vi "Dashboard Main.vi"() -> ()   [LabVIEW 2013]
uses:
  <vilib>/Utility/config.llb/NI_LVConfig.lvlib
  <vilib>/Utility/config.llb/Write Key (I32).vi
  <vilib>/Rock Robotics/WPI/Dashboard/WPI_DashboardLogging Global.vi
  <vilib>/Utility/config.llb/Write Key (String).vi
  <vilib>/ErrorRing/Error Ring.xnode
  <vilib>/Analysis/NI_AALBase.lvlib
  <vilib>/Analysis/baseanly.llb/Mean (DBL).vi
  Program Files (x86)/National Instruments/LabVIEW 2013/examples/FRC/Vision/2014 Target Detection/TargetType.ctl
panel:
  out "Image Message":string="Timeout in Camera Communications"
  in  "Rec Mode":enum32{"Stop", "Record", "Playback"}(radio)
  in  "Dashboard Tab":T1(tab)
  in  "Camera Settings":T2={"Frame Rate"=30, "Compression"=30, "Size"=1} {"Frame Rate" scale=1.0..30.0; "Size" items=["640x480", "320x240", "160x120"]}
  out "MotorSliders R":cluster{"MotorSlide1":dbl, "MotorSlide2":dbl} {"MotorSlide2" scale=-1.0..1.0 scale format="%#_2e"; "MotorSlide1" scale=-1.0..1.0 scale format="%#_2e"}
  out "MotorChart R":cluster{"Numeric":dbl, "Numeric":dbl}(graph)
  out "MotorSliders L":T3 {"MotorSlide4 2" scale=0.0..14.0 scale format="%#_2e"; "MotorSlide2" scale=-1.0..1.0 scale format="%#_2e"; "MotorSlide1" scale=-1.0..1.0 scale format="%#_2e"}
  out "MotorChart L":T4(graph)
  out "JS1 Z":dbl(slide) scale=-1.0..1.0 scale format="%#_2e"
  out "Joystick 1":cluster{"X":dbl, "Y":dbl}[](graph)
  out "JS Buttons 1":T5
  out "JS2 Z":dbl(slide) scale=-1.0..1.0 scale format="%#_2e"
  out "Joystick 2":cluster{"X":dbl, "Y":dbl}[](graph)
  out "JS Buttons 2":T5
  out "Mode":T6(ring)=enum."Auto Disabled"
  out "Camera IP":string
  in  "DB Camera Config":bool
  out "fps":dbl format="%#.1g"
  out "Mbps":dbl format="%#.1g"
  out "Mbps 2":bool
  in  "Ouput Image":enum16{"Original", "Overlay", "Binary"}(ring)
  in  "Color Components":T7={"Hue"={110.0, 142.0}, "Sat"={138.0, 255.0}, "Val"={139.0, 198.0}} {"Val" scale=0.0..255.0; "Sat" scale=0.0..255.0; "Hue" scale=0.0..255.0 scale format="%#_3g"}
  in  "Std Devs":cluster{"Hue":dbl, "Sat":dbl, "Val":dbl}={"Hue"=4.0, "Sat"=6.0, "Val"=4.0}
  in  "Area Size Limit %":dbl=0.06 format="%#_13g"
  in  "Score Cutoff":dbl(slide)=54.248366013071895 scale=0.0..100.0
  out "UltrasonicRF":dbl
  out "UltrasonicLF":dbl
  out "Glass Connected":bool
  out "High Pressure":dbl
  in  "Limit":dbl
  out "Encoder FR":dbl
  out "Encoder FL":dbl
  out "Encoder RR":dbl
  out "Encoder RL":dbl
  out "Low Pressure":dbl
  in  "P":dbl=1.0
  out "Motor Outputs":dbl[](graph)
  in  "I":dbl=0.01
  in  "D":dbl
  in  "Data To Glass Type":T8(ring)
  in  "Read To Shoot?":bool=TRUE
  in  "Autonomous Enabled":bool
  in  "Reset Score":bool
  out "Side Hot":enum16{"Hot", "Not Hot"}(ring)
  out "Chance Hot":dbl
  in  "Use Left/Right":enum16{"Left", "Right"}(ring)
  in  "Test Slider":dbl(slide) scale=0.0..100.0 scale format="%#_3g"
  in  "On/Off":bool caption="Solenoid"
  in  "Test Name":u16(ring) items=["Select the test to run...", "Example Test", "-------------------------------", "List of tests is built in robot code.", "Replace with your own automated tests."]
  in  "Test Tree":string(tree)
  in  "Motor":cluster{"Value":dbl, "Enable":bool} {"Value" scale=-1.0..1.0 scale format="%#_3g"}
  out "Progress":T9 {"Test Progress" scale=0.0..100.0}
  in  "Rev/Fwd":cluster{"Forward":bool, "Reverse":bool}
  in  "Test Ring":u16(ring) items=["Auto", "Fixed indoor", "Fixed outdoor 1", "Fixed outdoor 2", "Fixed fluorescent 1", "Fixed fluorescent 2", "Hold current"]
  out "Target Info":T11(array[cluster])
  out "Tree":string(tree)
  out "Camera Image":T12(plugin-control)
  in  "Enable":bool
  # "Left"
  # "Front"
  # "Right"
  # "Battery"
  # "(Move or Just Fire)"
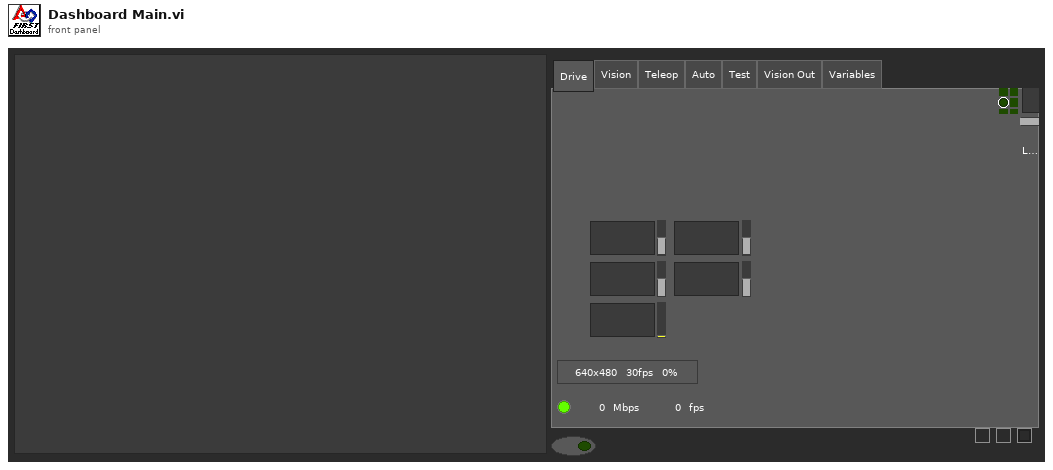
[diagram p1: front panel]
types:
  T1 = enum32{"Drive", "Vision", "Teleop", "Auto", "Test", "Vision Out", "Variables"}
  T2 = cluster{"Frame Rate":i32, "Compression":i32, "Size":u16}
  T3 = cluster{"MotorSlide1":dbl, "MotorSlide2":dbl, "MotorSlide4 2":dbl}
  T4 = cluster{"Numeric":dbl, "Numeric":dbl, "Battery":sgl}
  T5 = cluster{bool, bool, bool, bool, bool, bool, bool, bool, bool, bool, bool, bool}
  T6 = enum8{"Tele-Op Disabled", "Tele-Op Enabled", "Auto Disabled", "Auto Enabled", "Test Disabled", "Test Enabled", ""}
  T7 = cluster{"Hue":cluster{dbl, dbl}, "Sat":cluster{dbl, dbl}, "Val":cluster{dbl, dbl}}
  T8 = enum16{"Text (00)", "Shoot Status (01)", "Shoot Dist. (02)", "Pressure (03)", "Feed Dist. (04)", "Shutdown (99)"}
  T9 = cluster{"Test Progress":u8, "Test Progress Text":string}
  T10 = typedef "TargetType.ctl" = enum16{"Not Hot", "Hot"}
  T11 = cluster{"Scores":cluster{"Total":dbl, "Left":dbl, "Right":dbl, "Ratio":dbl, "Vertical":dbl, "index":i32, "State":T10}, "Verticals":cluster{"Horizontal?":bool, "Aspect Score":dbl, "Rect Score":dbl, cluster{"Left":dbl, "Top":dbl, "Right":dbl, "Bottom":dbl}, "Equiv H":dbl, "Equiv V":dbl}, "Horizontals":cluster{"Horizontal?":bool, "Aspect Score":dbl, "Rect Score":dbl, cluster{"Left":dbl, "Top":dbl, "Right":dbl, "Bottom":dbl}, "Equiv H":dbl, "Equiv V":dbl}, "Distance ft":dbl, "Center":cluster{"X":dbl, "Y":dbl}}[]
  T12 = typedef "IMAQ Image.ctl" = refnum<image>
  T13 = enum32{"Drive", "Operation", "Auto", "Test", "Checklist", "Variables"}
  T14 = typedef "Image Type" = u32
  T15 = cluster{"Digital Inputs":bool[], "Digital Outputs":bool[]}
  T16 = cluster{"Competition mode":bool, "Robot Link":bool, "Autonomous":bool, "Enabled":bool, "E-Stop":bool, "Simulated":bool, "TestMode":bool, "Docked Window":bool}
  T17 = cluster{"Boolean Array[0]":bool, "Boolean Array[1]":bool, "Boolean Array[2]":bool, "Boolean Array[3]":bool, "Boolean Array[4]":bool, "Boolean Array[5]":bool, "Boolean Array[6]":bool, "Boolean Array[7]":bool, "Boolean Array[8]":bool, "Boolean Array[9]":bool, "Boolean Array[10]":bool, "Boolean Array[11]":bool}
  T18 = typedef "NI_LVConfig.lvlib/Config Data RefNum.ctl" = refnum<k1>
  T19 = cluster{"Image Size":bool, "Image Type":bool, "Pixel Value":bool, "ROI Information":bool, "Zoom Factor":bool}
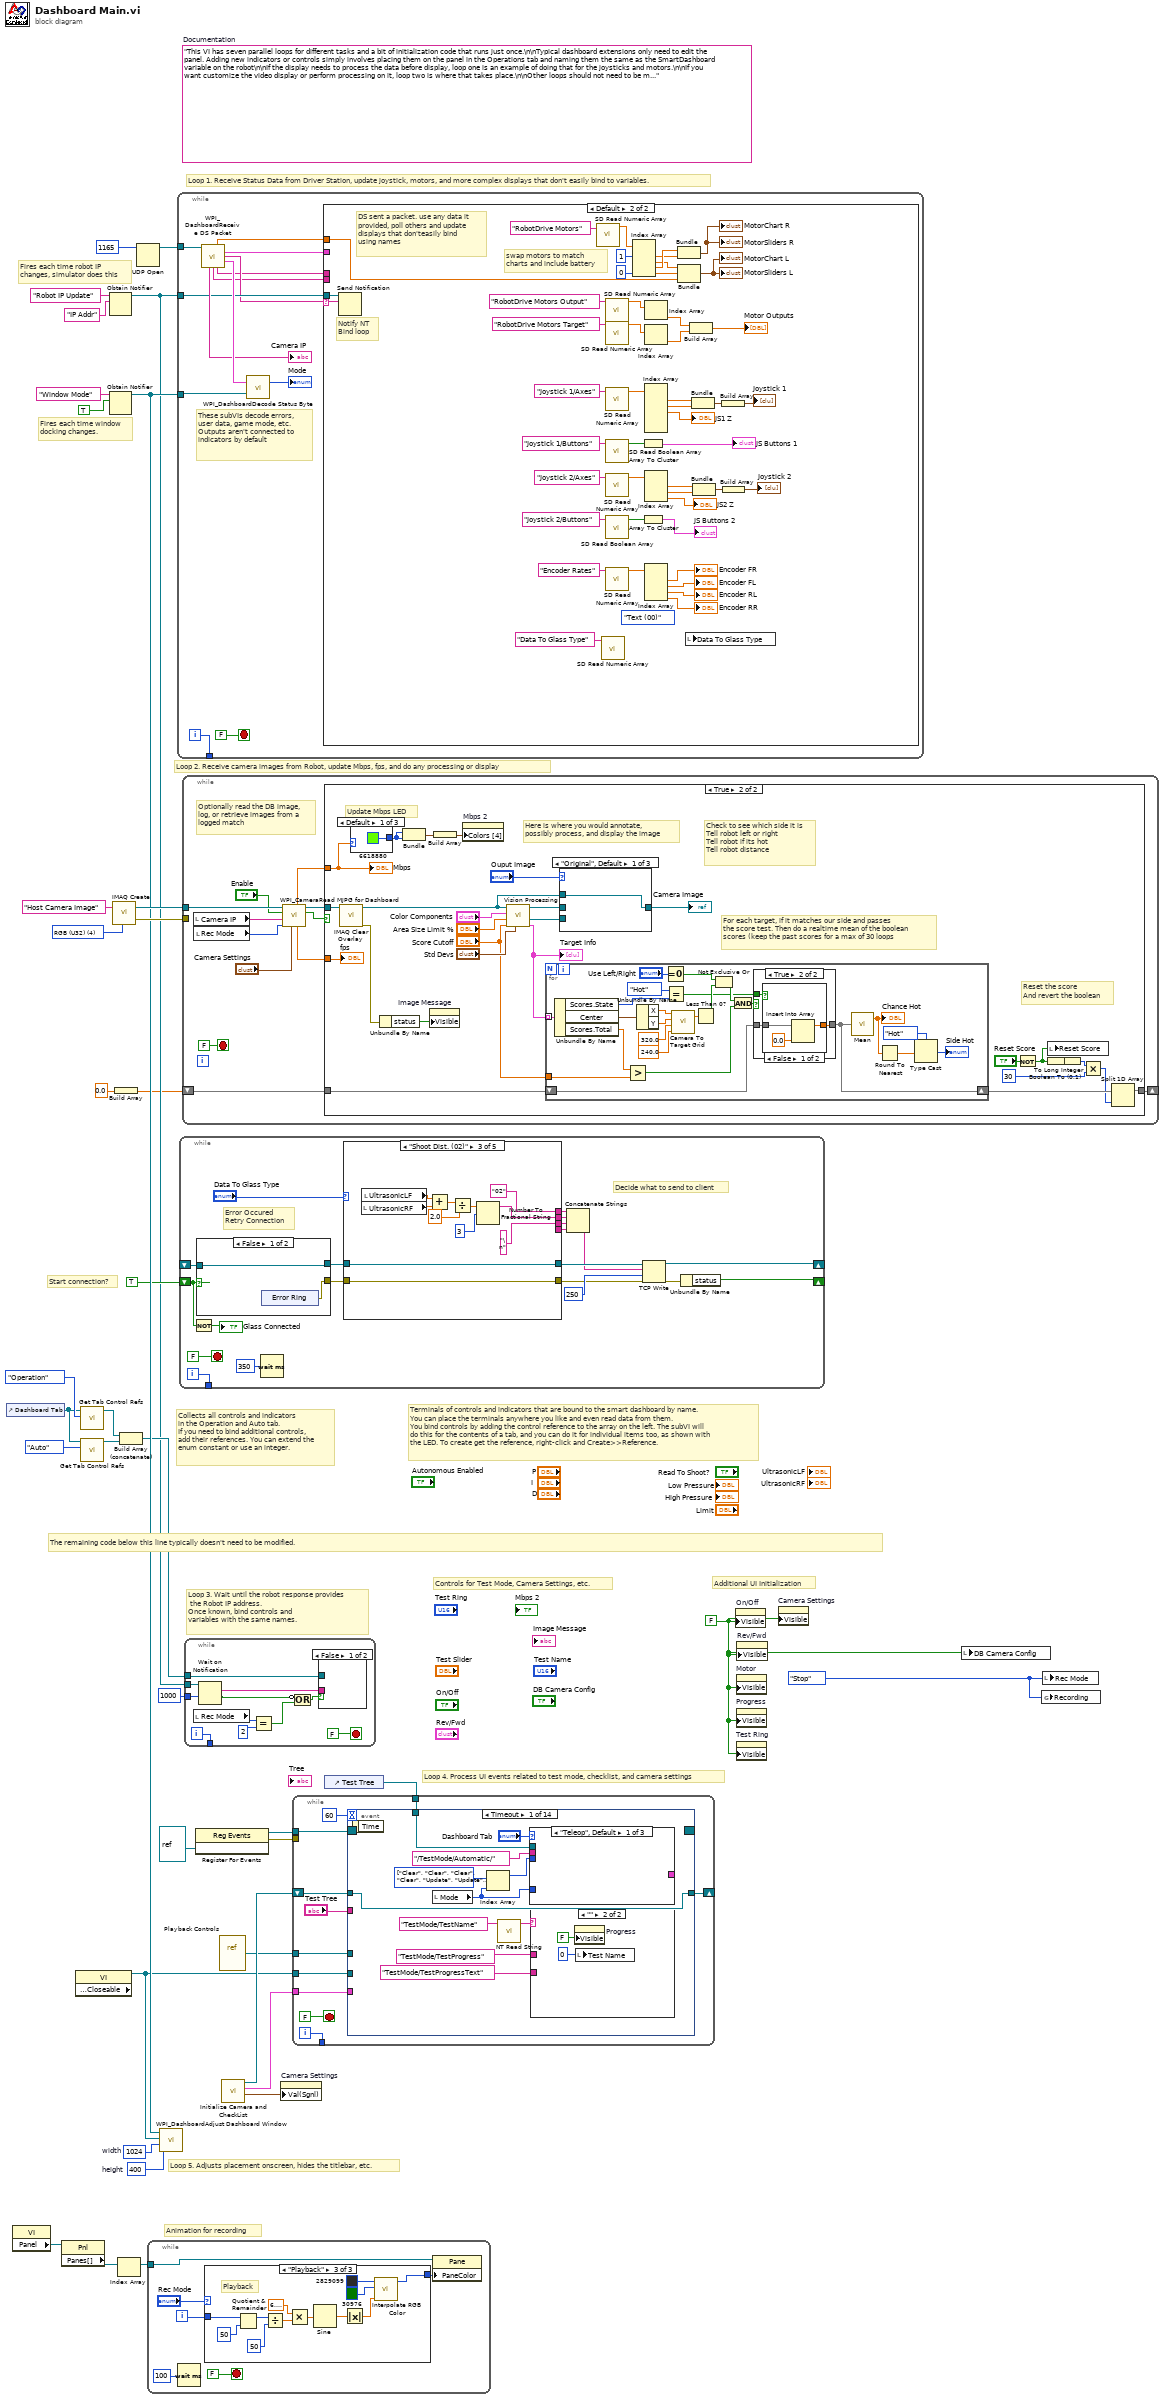
[diagram p0: block diagram]
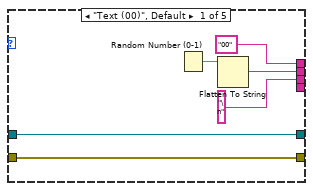
[diagram p2: hidden frame]
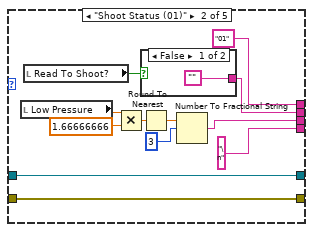
[diagram p3: hidden frame]
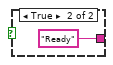
[diagram p4: hidden frame]
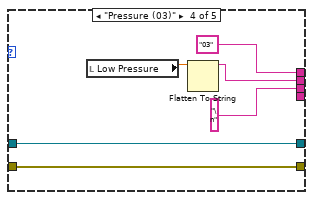
[diagram p5: hidden frame]
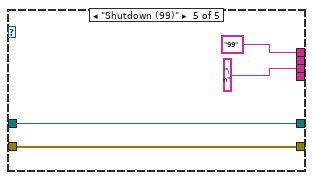
[diagram p6: hidden frame]
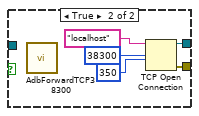
[diagram p7: hidden frame]
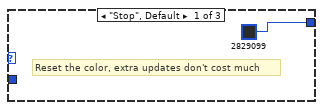
[diagram p8: hidden frame]
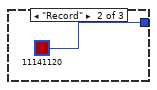
[diagram p9: hidden frame]
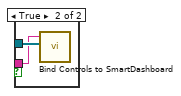
[diagram p10: hidden frame]
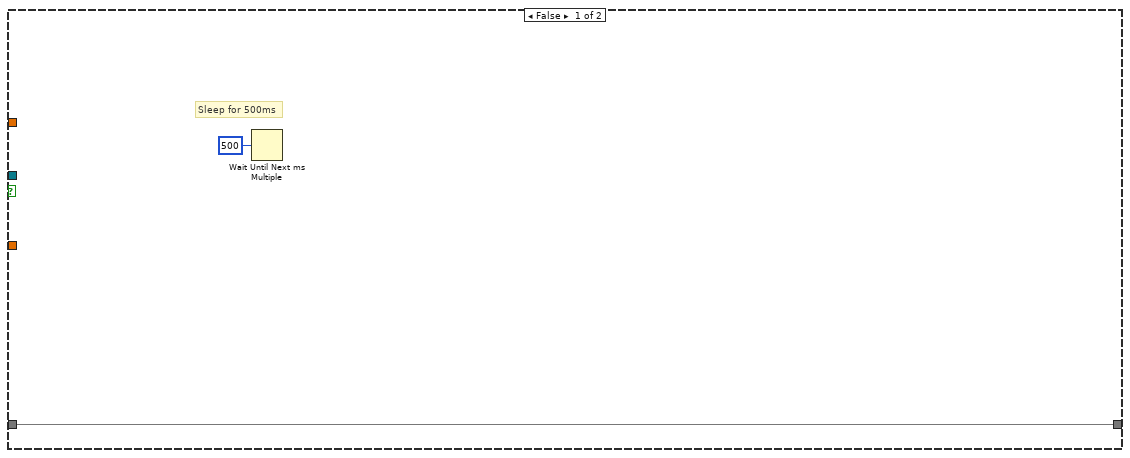
[diagram p11: hidden frame]
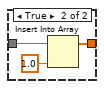
[diagram p13: hidden frame]
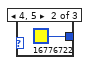
[diagram p16: hidden frame]
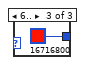
[diagram p17: hidden frame]
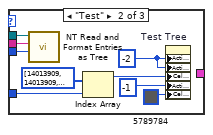
[diagram p18: hidden frame]
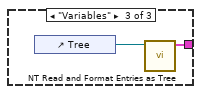
[diagram p19: hidden frame]
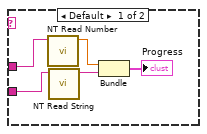
[diagram p20: hidden frame]
diagram:
  w11 = enum32{"Stop", "Record", "Playback"}."Stop" ("Rec Mode")
  w13 = 400  # height
  w14 = 1024  # width
  w27 = FALSE ("Visible")
  (unwired) "This VI has seven parallel loops for different tasks and a bit of initialization code that runs just once.\n\nTypical dashboard extensions only need to edit the panel. Adding new indicators or controls simply involves placing them on the panel in the Operations tab and naming them the same as the SmartDashboard variable on the robot\n\nIf the display needs to process the data before display, loop one is an example of doing that for the joysticks and motors.\n\nIf you want customize the video display or perform processing on it, loop two is where that takes place.\n\nOther loops should not need to be modified. They are pretty standard, and document the task they perform."  # Documentation
  w36 = T14 4 items=["Grayscale (U8)", "Grayscale (I16)", "Grayscale (SGL)", "Complex (CSG)", "RGB (U32)", "HSL (U32)", "RGB (U64)"] ("Image Type")
  # "Start connection?"
  # "Controls for Test Mode, Camera Settings, etc."
  # "Additional UI Initialization"
  # "Animation for recording"
  # "Fires each time robot IP\nchanges, simulator does this"
  # "Fires each time window\ndocking changes."
  # "Collects all controls and indicators\nin the Operation and Auto tab.\nIf you need to bind additional controls,\nadd their references. You can extend the\nenum constant or use an integer."
  # "The remaining code below this line typically doesn't need to be modified."
  # "Loop 4. Process UI events related to test mode, checklist, and camera settings"
  # "Terminals of controls and indicators that are bound to the smart dashboard by name.\nYou can place the terminals anywhere you like and even read data from them.\nYou bind controls by adding the control reference to the array on the left. The subVI will\ndo this for the contents of a tab, and you can do it for individual items too, as shown with\nthe LED. To create get the reference, right-click and Create>>Reference."
  # "Loop 3. Wait until the robot response provides\n the Robot IP address.\nOnce known, bind controls and\nvariables with the same names."
  # "Loop 5. Adjusts placement onscreen, hides the titlebar, etc."
  # "Loop 1. Receive Status Data from Driver Station, update joystick, motors, and more complex displays that don't easily bind to variables."
  # "Loop 2. Receive camera images from Robot, update Mbps, fps, and do any processing or display"
  n1 = control-ref of="Dashboard Tab"() -> (w9:refnum<vi>)
  n2 = property class="VI"() -> ("Panel"=w21:refnum<vi>)  [unwired: 2 in, 2 out]
  n3 = property class="Pnl"(reference=w21) -> ("Panes[]"=w22:refnum<vi>[])  [unwired: 1 in, 2 out]
  n4 = property class="VI" props=["Front Panel.Closeable"]() -> (reference out=w10:refnum<vi>)  [unwired: 2 in, 2 out]
  n5 = call <vilib>:"Get Tab Control Refs.vi"("Page Index"=T13."Operation" ("Dashboard Tab"), "TabControl in"=w9) -> ("ControlsOnPage"=w7:refnum<vi>[])  [unwired: 9 in]
  n6 = call <vilib>:"Get Tab Control Refs.vi"("Page Index"=T13."Auto" ("Dashboard Tab"), "TabControl in"=w9) -> ("ControlsOnPage"=w8:refnum<vi>[])  [unwired: 9 in]
  n7 = Obtain Notifier(name (unnamed)="Robot IP Update", notification data type="IP Addr" ("name (unnamed)")) -> (notifier out=w3:refnum<notifier>)  [unwired: 2 in, 2 out]
  n8 = Obtain Notifier(name (unnamed)="Window Mode", notification data type=TRUE) -> (notifier out=w12:refnum<notifier>)  [unwired: 2 in, 2 out]
  n9 = call "IMAQ Create"("Image Name"="Host Camera Image", "Image Type"=w36) -> ("New Image"=w34:T12, "error out"=w33:errorcluster)  [unwired: 2 in, 1 out]
  n10 = Build Array(0.0 ("element")) -> (w2:dbl[])
  n11 = Index Array(array=w22) -> (element=w20:refnum<vi>)  [unwired: 1 in]
  n12 = Build Array (concatenate)(w7, w8) -> (w6:refnum<vi>[])
  n13 = UDP Open(11:u16 1165 ("port")) -> (port=w37:refnum<k16>)  [unwired: 2 in, 4 out]
  n14 = while {
    tunnel: w20 -> [w40]
    i -> [w43]
    stop <- FALSE stop-if-true
    n15 = Wait (ms)(milliseconds to wait=u32 100) -> ()  [unwired: 1 out]
    n16 = case shown="\"Playback\"" "Rec Mode" {
      tunnel: w43 -> [_ _ w58]
      tunnel: [u32 2829099 ("Base Color") u32 11141120 ("Target Color") w47] -> w39
      frame "Stop", Default {
        # "Reset the color, extra updates don't cost much"
      }
      frame "Record" {
      }
      frame "Playback" {
        # "Playback"
        n17 = Quotient & Remainder(x=w58, y=u32 50 ("milliseconds to wait")) -> (x-y*floor(x/y)=w54:u32)  [unwired: 1 out]
        n18 = Divide(x=w54, y=u32 50 ("milliseconds to wait")) -> (x/y=w51:dbl)
        n19 = Multiply(x=6.283185307179586, y=w51) -> (x*y=w56:dbl)
        n20 = Sine(x=w56) -> (sin(x)=w55:dbl)
        n21 = Absolute Value(x=w55) -> (abs(x)=w48:dbl)
        n22 = call "Interpolate RGB Color.vi"("Proportion"=w48, "Target Color"=u32 30976, "Base Color"=u32 2829099) -> ("Result Color"=w47:u32)  [unwired: 8 in]
      }
    }
    n23 = property class="Pane"(reference=w40, "PaneColor"=w39) -> ()  [unwired: 1 in, 2 out]
  }
  n24 = call <vilib>:"WPI_DashboardAdjust Dashboard Window.vi"("height"=w13, "width"=w14, "reference in"=w10, "Notifier in"=w12) -> ()  [unwired: 8 in]
  n25 = while {
    tunnel: w37 -> [w69]
    tunnel: w3 -> [w64]
    tunnel: w12 -> [w68]
    tunnel: [w65] -> _
    i -> [w65]
    stop <- FALSE stop-if-true
    # "These subVIs decode errors, user data, game mode, etc.\nOutputs aren't connected to indicators by default"
    n26 = call <vilib>:"WPI_DashboardReceive DS Packet.vi"("Recv Socket"=w69) -> ("Battery"=w59:sgl, "Driver Station"=w60:T15, "Robot IP Address"=w63:string, "Status"=w70:T16, "Camera IP Address"=→"Camera IP":string, "Low Priority User Data"=w62:string, "High Priority User Data"=w61:string)  [unwired: 1 in, 7 out]
    n27 = call <vilib>:"WPI_DashboardDecode Status Byte.vi"("Window Mode Notifier"=w68, "Status"=w70) -> ("Mode"=→"Mode":T6)  [unwired: 1 out]
    n28 = case shown="Default" w63 {
      selector: w63 -> [_ w96]
      tunnel: w64 -> [_ w97]
      tunnel: w62 -> [_ _]
      tunnel: w61 -> [_ _]
      tunnel: w60 -> [_ _]
      tunnel: w59 -> [_ w95]
      frame "0.0.0.0" {
        # "DS not sending packets, or no robot exists yet.\nDon't poll the variables"
      }
      frame Default {
        (unwired) T8."Text (00)" ("Data To Glass Type")
        # "Notify NT\nBind loop"
        # "DS sent a packet. use any data it\nprovided, poll others and update\ndisplays that don'teasily bind\nusing names"
        # "swap motors to match\ncharts and include battery"
        n29 = Send Notification(notification=w96, notifier=w97) -> ()  [unwired: 1 in, 2 out]
        n30 = call <vilib>:"SD Read Numeric Array.vi"("Name"="RobotDrive Motors") -> ("Numeric Array"=w94:dbl[])  [unwired: 8 in, 2 out]
        n31 = call <vilib>:"SD Read Numeric Array.vi"("Name"="Data To Glass Type") -> ()  [unwired: 8 in, 3 out]
        n32 = call <vilib>:"SD Read Numeric Array.vi"("Name"="RobotDrive Motors Output") -> ("Numeric Array"=w82:dbl[])  [unwired: 8 in, 2 out]
        n33 = call <vilib>:"SD Read Numeric Array.vi"("Name"="RobotDrive Motors Target") -> ("Numeric Array"=w80:dbl[])  [unwired: 8 in, 2 out]
        n34 = call <vilib>:"SD Read Numeric Array.vi"("Name"="Joystick 1/Axes") -> ("Numeric Array"=w113:dbl[])  [unwired: 8 in, 2 out]
        n35 = call <vilib>:"SD Read Boolean Array.vi"("Name"="Joystick 1/Buttons") -> ("Boolean Array"=w115:bool[])  [unwired: 8 in, 2 out]
        n36 = call <vilib>:"SD Read Numeric Array.vi"("Name"="Joystick 2/Axes") -> ("Numeric Array"=w107:dbl[])  [unwired: 8 in, 2 out]
        n37 = call <vilib>:"SD Read Boolean Array.vi"("Name"="Joystick 2/Buttons") -> ("Boolean Array"=w106:bool[])  [unwired: 8 in, 2 out]
        n38 = call <vilib>:"SD Read Numeric Array.vi"("Name"="Encoder Rates") -> ("Numeric Array"=w75:dbl[])  [unwired: 8 in, 2 out]
        n39 = Index Array(array=w94, index #1=1, index #4=0) -> (element #1=w90:dbl, element #2=w89:dbl, element #3=w91:dbl, element #4=w86:dbl)  [unwired: 2 in]
        n40 = Array To Cluster(array=w115) -> (cluster=→"JS Buttons 1":T17)
        n41 = Array To Cluster(array=w106) -> (cluster=→"JS Buttons 2":T17)
        n42 = Index Array(array=w82) -> (element=w81:dbl)  [unwired: 1 in]
        n43 = Index Array(array=w80) -> (element=w74:dbl)  [unwired: 1 in]
        n44 = Index Array(array=w113) -> (element #1=w110:dbl, element #2=w111:dbl, element #3=→"JS1 Z":dbl)  [unwired: 6 in, 3 out]
        n45 = Index Array(array=w107) -> (element #1=w102:dbl, element #2=w101:dbl, element #3=→"JS2 Z":dbl)  [unwired: 3 in]
        n46 = Index Array(array=w75) -> (element #1=→"Encoder FR":dbl, element #2=→"Encoder FL":dbl, element #3=→"Encoder RL":dbl, element #4=→"Encoder RR":dbl)  [unwired: 4 in]
        n47 = Bundle("Numeric"=w91, "Numeric"=w90) -> (→"MotorChart R" →"MotorSliders R":cluster{"Numeric":dbl, "Numeric":dbl})  [unwired: 1 in]
        n48 = Bundle("Numeric"=w89, "Numeric"=w86, "Battery"=w95) -> (→"MotorChart L" →"MotorSliders L":T4)  [unwired: 1 in]
        n49 = local read "Data To Glass Type"() -> ()  [unwired: 1 in]
        n50 = Build Array(w81, w74) -> (→"Motor Outputs":dbl[])
        n51 = Bundle("Numeric"=w110, "Numeric"=w111) -> (w109:cluster{"Numeric":dbl, "Numeric":dbl})  [unwired: 1 in]
        n52 = Bundle("Numeric"=w102, "Numeric"=w101) -> (w103:cluster{"Numeric":dbl, "Numeric":dbl})  [unwired: 1 in]
        n53 = Build Array(w109) -> (→"Joystick 1":cluster{"Numeric":dbl, "Numeric":dbl}[])
        n54 = Build Array(w103) -> (→"Joystick 2":cluster{"Numeric":dbl, "Numeric":dbl}[])
      }
    }
  }
  n55 = while {
    tunnel: [w137] -> _
    shift-right: [w134] -> _
    shift-left: TRUE ("status") -> [w120]
    shift-right: [w133] -> _
    shift-left: _ -> [w132]
    i -> [w137]
    stop <- FALSE stop-if-true
    # "Decide what to send to client"
    # "Error Occured \nRetry Connection"
    n56 = Not(x=w120) -> (.not. x?=→"Glass Connected":bool)
    n57 = case shown="False" w120 {
      tunnel: [w181 w184] -> w127
      tunnel: [w180 w183] -> w129
      tunnel: w132 -> [w181 _]
      frame False {
        n58 = xnode "Error Ring"() -> ("error out"=w180:errorcluster)
      }
      frame True {
        n59 = call "AdbForwardTCP38300.vi"() -> ()  [unwired: 12 in]
        n60 = TCP Open Connection(address="localhost", remote port or service name=u16 38300, timeout ms (60000)=350) -> (connection ID=w184:refnum<k5>, error out=w183:errorcluster)  [unwired: 2 in]
      }
    }
    n61 = Wait (ms)(milliseconds to wait=u32 350) -> ()  [unwired: 1 out]
    n62 = case shown="\"Shoot Dist. (02)\"" "Data To Glass Type" {
      tunnel: [w143 w155 w163 w174 w178] -> w128
      tunnel: w129 -> [w143 w155 w163 w174 w178]
      tunnel: w127 -> [w142 w156 w160 w175 w179]
      tunnel: [w142 w156 w160 w175 w179] -> w126
      tunnel: ["\n" ("string") w146 "\n" ("string") "\n" ("string") "\n" ("string")] -> w124
      tunnel: ["00" ("string") "01" ("string") "02" ("string") "03" ("string") "99" ("string")] -> w123
      tunnel: [w140 w152 w162 w171 _] -> w122
      tunnel: [_ "\n" ("string") _ _ _] -> w119
      frame "Text (00)", Default {
        n63 = Random Number (0-1)() -> (number: 0 to 1=w144:dbl)
        n64 = Flatten To String(anything=w144) -> (data string=w140:string)  [unwired: 3 in, 2 out]
      }
      frame "Shoot Status (01)" {
        n65 = local read "Low Pressure"() -> (w150:dbl)
        n66 = local read "Read To Shoot?"() -> (w154:bool)
        n67 = Multiply(x=w150, y=1.66666666) -> (x*y=w149:dbl)
        n68 = case shown="False" w154 {
          tunnel: ["" "Ready"] -> w152
          frame False {
          }
          frame True {
          }
        }
        n69 = Round To Nearest(number=w149) -> (nearest integer value=w147:dbl)
        n70 = Number To Fractional String(number=w147, width (-)=i16 3) -> (F-format string=w146:string)  [unwired: 2 in]
      }
      frame "Shoot Dist. (02)" {
        n71 = local read "UltrasonicRF"() -> (w168:dbl)
        n72 = local read "UltrasonicLF"() -> (w169:dbl)
        n73 = Add(x=w169, y=w168) -> (x+y=w167:dbl)
        n74 = Divide(x=w167, y=2.0) -> (x/y=w161:dbl)
        n75 = Number To Fractional String(number=w161, width (-)=i16 3) -> (F-format string=w162:string)  [unwired: 2 in]
      }
      frame "Pressure (03)" {
        n76 = local read "Low Pressure"() -> (w173:dbl)
        n77 = Flatten To String(anything=w173) -> (data string=w171:string)  [unwired: 3 in, 2 out]
      }
      frame "Shutdown (99)" {
      }
    }
    n78 = Concatenate Strings(w123, w122, w124, w119) -> (w125:string)
    n79 = TCP Write(connection ID=w126, data in=w125, error in (no error)=w128, 9:250 ("timeout ms (25000)")) -> (connection ID out=w133:refnum<k5>, error out=w135:errorcluster)  [unwired: 1 out]
    n80 = Unbundle By Name(w135) -> ("status"=w134:bool)
  }
  n81 = while {
    tunnel: w34 -> [w198]
    tunnel: w33 -> [_]
    shift-right: [w188] -> _
    shift-left: w2 -> [w189]
    stop <- FALSE stop-if-true
    # "Optionally read the DB image,\nlog, or retrieve images from a\nlogged match"
    n82 = local read "Camera IP"() -> (w191:string)
    n83 = local read "Rec Mode"() -> (w190:enum32{"Stop", "Record", "Playback"})
    n84 = call <vilib>:"WPI_CameraRead MJPG for Dashboard.vi"("Camera Settings"="Camera Settings", "Rec Mode"=w190, "Camera IP"=w191, "Enable"="Enable", "Refnum in"=w198) -> ("Active"=w195:bool, "Refnum out"=w197:T12, "FPS"=w194:dbl, "Bandwidth (Mbps)"=w193:dbl)  [unwired: 3 in]
    n85 = case shown="True" w195 {
      tunnel: w197 -> [_ w223]
      tunnel: w193 -> [_ w222]
      tunnel: w194 -> [_ w221]
      tunnel: w189 -> [w200 w210]
      tunnel: [w200 w208] -> w188
      frame False {
        # "Sleep for 500ms"
        n86 = Wait Until Next ms Multiple(millisecond multiple=u32 500) -> ()  [unwired: 1 out]
      }
      frame True {
        # "Reset the score\nAnd revert the boolean"
        # "For each target, if it matches our side and passes\nthe score test. Then do a realtime mean of the boolean\nscores (keep the past scores for a max of 30 loops"
        # "Check to see which side it is\nTell robot left or right\nTell robot if its hot\nTell robot distance"
        # "Here is where you would annotate,\npossibly process, and display the image"
        # "Update Mbps LED"
        n87 = call "IMAQ Clear Overlay"("Image"=w223) -> ("error out"=w227:errorcluster, "Image Out"=w213:T12)  [unwired: 2 in, 7 out]
        n88 = case shown="Default" w222 {
          tunnel: [u32 6618880 ("Color Box") u32 16776722 ("Color Box") u32 16716800 ("Color Box")] -> w224
          frame Default {
          }
          frame 4, 5 {
          }
          frame 6.. {
          }
        }
        n89 = Unbundle By Name(w227) -> ("status"=w228:bool)
        n90 = Bundle("Color Box"=w224, "Color Box"=w224) -> (w226:cluster{"Color Box":u32, "Color Box":u32})  [unwired: 1 out]
        n91 = property on="Image Message" class="Str"("Visible"=w228) -> ()  [unwired: 2 in, 2 out]
        n92 = Build Array(w226) -> (w225:cluster{"Color Box":u32, "Color Box":u32}[])
        n93 = property on="Mbps 2" class="Bool (strict)"("Colors [4]"=w225) -> ()  [unwired: 2 in, 2 out]
        n94 = call "Vision Processing.vi"("Std Devs"="Std Devs", "Score Cutoff"="Score Cutoff", "Area Size Limit %"="Area Size Limit %", "Color Components"="Color Components", "Image In"=w213) -> ("Target Info"=w212:T11, "Mask"=w214:T12, "Image Out"=w215:T12)  [unwired: 4 in]
        "Target Info" <- w212
        n95 = for {
          tunnel: w212 -> [w251] mode=indexing
          tunnel: "Score Cutoff" -> [w239]
          shift-right: [w229] -> w209
          shift-left: w210 -> [w234]
          n96 = Unbundle By Name(w251) -> ("Scores.State"=w245:T10, "Center"=w252:cluster{"X":dbl, "Y":dbl}, "Scores.Total"=w240:dbl)
          n97 = Greater?(x=w240, y=w239) -> (0:w232:bool)
          n98 = Unbundle By Name(w252) -> ("X"=w250:dbl, "Y"=w249:dbl)
          n99 = Equal To 0?(x="Use Left/Right") -> (x = 0?=w242:bool)
          n100 = Equal?(x=TargetType."Hot", y=w245) -> (x = y?=w230:bool)
          n101 = call "Camera To Target Grid.vi"("Height"=240.0, "Width"=320.0, "CY"=w249, "CX"=w250) -> ("X'"=w247:dbl)  [unwired: 1 out]
          n102 = Less Than 0?(x=w247) -> (x < 0?=w243:bool)
          n103 = Not Exclusive Or(1:w243, 2:w242) -> (0:w231:bool)
          n104 = And(x=w231, y=w232) -> (x .and. y?=w233:bool)
          n105 = case shown="True" w233 {
            tunnel: w234 -> [w253 w256]
            tunnel: [w253 w255] -> w229
            tunnel: w230 -> [_ w254]
            frame False {
            }
            frame True {
              n106 = case shown="False" w254 {
                tunnel: w256 -> [w258 w262]
                tunnel: [w257 w260] -> w255
                frame False {
                  n107 = Insert Into Array(array=w258, new element=0.0 ("new element/subarray")) -> (w257:dbl[])  [unwired: 1 in]
                }
                frame True {
                  n108 = Insert Into Array(array=w262, new element=1.0 ("new element/subarray")) -> (w260:dbl[])  [unwired: 1 in]
                }
              }
            }
          }
          n109 = call-poly <vilib>:"Mean.vi"("X"=w229) -> ("mean"=w238:dbl)  [unwired: 1 out]
          "Chance Hot" <- w238
          n110 = Round To Nearest(number=w238) -> (nearest integer value=w235:dbl)
          n111 = Type Cast(type=enum16{"Hot", "Not Hot"}."Hot" ("Side Hot"), x=w235) -> (*(type *) &x=→"Side Hot":enum16{"Hot", "Not Hot"})
        }
        n112 = case shown="\"Original\", Default" "Ouput Image" {
          tunnel: [w263 w264 w265] -> w216
          tunnel: w215 -> [_ w264 _]
          tunnel: w214 -> [_ _ w265]
          tunnel: w213 -> [w263 _ _]
          frame "Original", Default {
          }
          frame "Overlay" {
          }
          frame "Binary" {
          }
        }
        "Camera Image" <- w216
        n113 = Not(x="Reset Score") -> (.not. x?=w202:bool)
        n114 = Boolean To (0,1)(Boolean=w202) -> (0, 1=w205:i16)
        n115 = local write "Reset Score"(w202) -> ()
        n116 = To Long Integer(number=w205) -> (32bit integer=w204:i32)
        n117 = Multiply(x=w204, y=30 ("index")) -> (x*y=w203:i32)
        n118 = Split 1D Array(array=w209, index=w203) -> (first subarray=w208:dbl[])  [unwired: 1 out]
        "Mbps" <- w222
        "fps" <- w221
      }
    }
  }
  n119 = while {
    tunnel: w6 -> [w279]
    tunnel: w3 -> [w277]
    tunnel: [w275] -> _
    tunnel: u32 1000 ("milliseconds to wait") -> [w274]
    i -> [w275]
    stop <- FALSE stop-if-true
    n120 = local read "Rec Mode"() -> (w270:enum32{"Stop", "Record", "Playback"})
    n121 = Wait on Notification(notifier=w277, timeout in ms (-1)=w274) -> (notification=w276:string, timed out?=w272:bool)  [unwired: 2 in, 2 out]
    n122 = Equal?(x=w270, y=u16 2 ("Rec Mode")) -> (x = y?=w271:bool)
    n123 = Compound Arithmetic op=OR(invert w272, w271) -> (w273:bool)
    n124 = case shown="False" w273 {
      tunnel: w279 -> [_ w281]
      tunnel: w276 -> [_ w280]
      frame False {
      }
      frame True {
        n125 = call <vilib>:"Bind Controls to SmartDashboard.vi"("Bound Control Refs"=w281, "Server IP Address"=w280) -> ()  [unwired: 10 in]
      }
    }
  }
  n126 = register-events(refnum<vi> refnum) -> (reference out=w18:refnum<event-registration>, error out=w17:errorcluster)  [unwired: 2 in]
  n127 = vi-ref "Playback Controls.vi"() -> (w19:refnum<vi>)
  n128 = call "Initialize Camera and CheckList.vi"() -> ("Cluster"=w25:cluster{"value":i32, "value":i32, "index":i32}, "Array"=w26:cluster{string[]}[], "File Refnum"=w24:T18)  [unwired: 9 in]
  n129 = property on="Camera Settings" class="Clust (strict)"("Val(Sgnl)"=w25) -> ()  [unwired: 2 in, 2 out]
  n130 = control-ref of="Test Tree"() -> (w23:refnum<vi>)
  n131 = while {
    tunnel: w26 -> [w289]
    shift-right: [w288] -> _
    shift-left: w24 -> [w287]
    tunnel: [w286] -> _
    tunnel: w23 -> [w285]
    tunnel: w19 -> [w284]
    tunnel: w18 -> [w283]
    tunnel: w17 -> [_]
    tunnel: w10 -> [w282]
    i -> [w286]
    stop <- FALSE stop-if-true
    n132 = event shown="[0] Timeout" {
      selector: w283 -> [_ _ _ _ _ _ _ _ _ _ _ _ _ _]
      dyn-events: [_ _ _ _ _ _ _ _ _ _ _ w503 _ _] -> _
      timeout: u32 60 ("milliseconds to wait") -> [_ _ _ _ _ _ _ _ _ _ _ _ _ _]
      tunnel: w285 -> [w299 _ _ _ _ _ _ _ _ _ _ _ _ _]
      tunnel: "Test Tree" -> [_ _ _ _ _ _ w472 w480 w482 w486 w494 _ _ _]
      tunnel: w289 -> [_ w323 _ _ w436 w466 _ _ _ _ _ _ _ _]
      tunnel: [w293 w322 w421 w426 w435 w459 w471 w478 w481 w485 w493 w505 w519 w520] -> w288
      tunnel: w287 -> [w293 w322 w421 w426 w434 w459 w471 w478 w481 w485 w493 w505 w519 w520]
      tunnel: w284 -> [_ _ _ _ _ _ _ _ _ _ _ w506 _ w523]
      tunnel: w282 -> [_ _ _ _ _ _ _ _ _ _ _ w501 _ _]
      event Timeout {
        w298 = enum16{"Update", "Clear"}[] [enum."Clear", enum."Clear", enum."Clear", enum."Clear", enum."Update", enum."Update", enum."Clear"] items=["Update", "Clear"]
        n133 = event-data() -> ()  [unwired: 1 in, 1 out]
        n134 = local read "Mode"() -> (w296:T6)
        n135 = Index Array(array=w298, index=w296) -> (element=w297:enum16{"Update", "Clear"})
        n136 = call <vilib>:"NT Read String.vi"("Name"="TestMode/TestName") -> ("String"=w302:string)  [unwired: 9 in, 1 out]
        n137 = case shown="\"Teleop\", Default" "Dashboard Tab" {
          tunnel: w299 -> [_ w312 _]
          tunnel: "/TestMode/Automatic/" ("Name Pattern") -> [_ w311 _]
          tunnel: w297 -> [_ w310 _]
          tunnel: w296 -> [_ w308 _]
          tunnel: [_ _ w314] -> _
          frame "Teleop", Default {
          }
          frame "Test" {
            w307 = -2 ("Active Item:Row Number")
            n138 = call <vilib>:"NT Read and Format Entries as Tree.vi"("Operation"=w310, "Name Pattern"=w311, "Tree Refnum"=w312) -> ()  [unwired: 7 in, 2 out]
            n139 = Index Array(array=u32[] [14013909, 14013909, 14013909, 14013909, 14013909, 16777215, 14013909], index=w308) -> (element=w306:u32)
            n140 = property on="Test Tree" class="Tree (strict)"("Active Item Row Number"=w307, "ActiveColNum"=w307, "CellBG"=w306, "Active Item Row Number"=-1 ("Active Item:Row Number"), "CellBG"=u32 5789784 ("Color Box")) -> ()  [unwired: 2 in, 2 out]
          }
          frame "Variables" {
            n141 = control-ref of="Tree"() -> (w313:refnum<vi>)
            n142 = call <vilib>:"NT Read and Format Entries as Tree.vi"("Tree Refnum"=w313) -> ("Formatted Strings"=w314:cluster{"Name":string, "Value":string}[])  [unwired: 9 in, 1 out]
          }
        }
        n143 = case shown="\"\"" w302 {
          tunnel: "TestMode/TestProgress" ("Name") -> [w316 _]
          tunnel: "TestMode/TestProgressText" ("Name") -> [w315 _]
          frame Default {
            n144 = call <vilib>:"NT Read Number.vi"("Name"=w316) -> ("Numeric"=w317:dbl)  [unwired: 9 in, 1 out]
            n145 = call <vilib>:"NT Read String.vi"("Name"=w315) -> ("String"=w318:string)  [unwired: 9 in, 1 out]
            n146 = Bundle("Numeric"=w317, "String"=w318) -> (→"Progress":cluster{"Numeric":dbl, "String":string})  [unwired: 1 in]
          }
          frame "" {
            n147 = property on="Progress" class="Clust (strict)"("Visible"=FALSE) -> ()  [unwired: 2 in, 2 out]
            n148 = local write "Test Name"(u16 0) -> ()
          }
        }
      }
      event "Test Tree": Value Change {
        # "Show appropriate\ncontrols"
        n149 = event-data() -> ("CtlRef"=w326:refnum<vi>, "NewVal"=w324:string)  [unwired: 1 in]
        n150 = call <vilib>:"WPI_UtilitiesGetTreeIOName.vi"("NewVal"=w324, "TreeControl in"=w326) -> ("I/O Name"=w327:string)  [unwired: 9 in]
        n151 = case shown="\"Camera\"" w327 {
          selector: w327 -> [_ w334 _ w352 w361 _]
          tunnel: w324 -> [_ _ w349 w351 _ w368]
          tunnel: w323 -> [_ _ _ _ _ w367]
          frame Default {
            w329 = FALSE ("Visible")
            w328 = FALSE ("Visible")
            n152 = property on="Motor" class="Clust (strict)"("Visible"=w328) -> ()  [unwired: 2 in, 2 out]
            n153 = property on="Test Ring" class="Ring (strict)"("Visible"=w328) -> ()  [unwired: 2 in, 2 out]
            n154 = property on="Rev/Fwd" class="Clust (strict)"("Visible"=w329) -> ()  [unwired: 2 in, 2 out]
            n155 = property on="On/Off" class="Bool (strict)"("Visible"=w329) -> ()  [unwired: 2 in, 2 out]
            n156 = property on="Test Slider" class="Slide (strict)"("Visible"=w329) -> ()  [unwired: 2 in, 2 out]
          }
          frame "Motor", "PWM" {
            w335 = FALSE ("Visible")
            n157 = case shown="\"Motor\", Default" w334 {
              tunnel: [1.0 ("Value") -1.0 ("Value")] -> w333
              tunnel: [255.0 ("Value") 1.0 ("Value")] -> w332
              tunnel: [128.0 ("Value") 0.0 ("Value")] -> w331
              tunnel: [64.0 ("Value") 0.5 ("Value")] -> w330
              frame "PWM" {
              }
              frame "Motor", Default {
              }
            }
            n158 = property on="Motor" class="Clust (strict)"("Visible"=TRUE) -> ()  [unwired: 2 in, 2 out]
            n159 = property on="Value" class="Slide (strict)"("Value"=w331, "Scale.Minimum"=w333, "Scale.Maximum"=w332, "Scale.Increment"=w330) -> ()  [unwired: 2 in, 2 out]
            n160 = property on="On/Off" class="Bool (strict)"("Visible"=w335) -> ()  [unwired: 2 in, 2 out]
            n161 = property on="Test Slider" class="Slide (strict)"("Visible"=w335) -> ()  [unwired: 2 in, 2 out]
            n162 = property on="Test Ring" class="Ring (strict)"("Visible"=w335) -> ()  [unwired: 2 in, 2 out]
            n163 = property on="Rev/Fwd" class="Clust (strict)"("Visible"=w335) -> ()  [unwired: 2 in, 2 out]
          }
          frame "Servo" {
            w347 = FALSE ("Visible")
            n164 = call <vilib>:"NT Read Number.vi"("Name"=w349) -> ("Numeric"=w348:dbl)  [unwired: 9 in, 1 out]
            n165 = property on="Test Slider" class="Slide (strict)"("Visible"=TRUE, "Scale.Maximum"=170.0 ("Scale.Range:Maximum")) -> ()  [unwired: 2 in, 2 out]
            n166 = local write "Test Slider"(w348) -> ()
            n167 = property on="Motor" class="Clust (strict)"("Visible"=w347) -> ()  [unwired: 2 in, 2 out]
            n168 = property on="Rev/Fwd" class="Clust (strict)"("Visible"=w347) -> ()  [unwired: 2 in, 2 out]
            n169 = property on="On/Off" class="Bool (strict)"("Visible"=w347) -> ()  [unwired: 2 in, 2 out]
            n170 = property on="Test Ring" class="Ring (strict)"("Visible"=w347) -> ()  [unwired: 2 in, 2 out]
          }
          frame "Relay", "Solenoid" {
            w350 = FALSE ("Visible")
            n171 = property on="Motor" class="Clust (strict)"("Visible"=w350) -> ()  [unwired: 2 in, 2 out]
            n172 = property on="Test Slider" class="Slide (strict)"("Visible"=w350) -> ()  [unwired: 2 in, 2 out]
            n173 = Search and Replace String(input string=w351, search string="/Value  **", replace string="/Direction") -> (result string=w357:string)  [unwired: 5 in, 3 out]
            n174 = property on="Test Ring" class="Ring (strict)"("Visible"=w350) -> ()  [unwired: 2 in, 2 out]
            n175 = call <vilib>:"NT Read String.vi"("Name"=w357) -> ("String"=w355:string)  [unwired: 9 in, 1 out]
            n176 = Equal?(x="Both directions", y=w355) -> (x = y?=w353:bool)
            n177 = Not(x=w353) -> (.not. x?=w354:bool)
            n178 = property on="Rev/Fwd" class="Clust (strict)"("Visible"=w353) -> ()  [unwired: 2 in, 2 out]
            n179 = property on="On/Off" class="Bool (strict)"("Visible"=w354, "Caption.Text"=w352) -> ()  [unwired: 2 in, 2 out]
          }
          frame "Compressor", "Digital Out" {
            w360 = FALSE ("Visible")
            # "Get direction and finish"
            n180 = property on="Motor" class="Clust (strict)"("Visible"=w360) -> ()  [unwired: 2 in, 2 out]
            n181 = property on="Test Slider" class="Slide (strict)"("Visible"=w360) -> ()  [unwired: 2 in, 2 out]
            n182 = property on="Test Ring" class="Ring (strict)"("Visible"=w360) -> ()  [unwired: 2 in, 2 out]
            n183 = property on="On/Off" class="Bool (strict)"("Visible"=TRUE, "Caption.Text"=w361) -> ()  [unwired: 2 in, 2 out]
            n184 = property on="Rev/Fwd" class="Clust (strict)"("Visible"=FALSE) -> ()  [unwired: 2 in, 2 out]
          }
          frame "Camera" {
            n185 = call <vilib>:"Get Last Path Segment.vi"("String in"=w368) -> ("String out"=w369:string)  [unwired: 10 in]
            n186 = property on="On/Off" class="Bool (strict)"("Visible"=FALSE) -> ()  [unwired: 2 in, 2 out]
            n187 = property on="Motor" class="Clust (strict)"("Visible"=FALSE) -> ()  [unwired: 2 in, 2 out]
            n188 = property on="Rev/Fwd" class="Clust (strict)"("Visible"=FALSE) -> ()  [unwired: 2 in, 2 out]
            n189 = case shown="\"White Balance  **\"" w369 {
              tunnel: w368 -> [w375 w384 w393 w402 w411 _ w417]
              tunnel: w367 -> [w373 w381 w390 w399 w408 _ _]
              frame "Size  **" {
                n190 = Index Array(array=w373) -> (element=w372:cluster{string[]})  [unwired: 1 in]
                n191 = call <vilib>:"NT Read String.vi"("Name"=w375) -> ("String"=w374:string)  [unwired: 9 in, 1 out]
                n192 = Unbundle(w372) -> (w370:string[])
                n193 = Match First String(2:w370, 3:w374) -> (0:w371:i32)  [unwired: 1 out]
                n194 = property on="Test Ring" class="Ring (strict)"("Value"=w371, "Strings []"=w370) -> ()  [unwired: 2 in, 2 out]
                n195 = property on="Test Ring" class="Ring (strict)"("Visible"=TRUE) -> ()  [unwired: 2 in, 2 out]
                n196 = property on="Test Slider" class="Slide (strict)"("Visible"=FALSE) -> ()  [unwired: 2 in, 2 out]
              }
              frame "White Balance  **" {
                n197 = Index Array(array=w381, index=1) -> (element=w382:cluster{string[]})
                n198 = call <vilib>:"NT Read String.vi"("Name"=w384) -> ("String"=w383:string)  [unwired: 9 in, 1 out]
                n199 = Unbundle(w382) -> (w379:string[])
                n200 = Match First String(2:w379, 3:w383) -> (0:w378:i32)  [unwired: 1 out]
                n201 = property on="Test Ring" class="Ring (strict)"("Value"=w378, "Strings []"=w379) -> ()  [unwired: 2 in, 2 out]
                n202 = property on="Test Ring" class="Ring (strict)"("Visible"=TRUE) -> ()  [unwired: 2 in, 2 out]
                n203 = property on="Test Slider" class="Slide (strict)"("Visible"=FALSE) -> ()  [unwired: 2 in, 2 out]
              }
              frame "Exposure  **" {
                n204 = Index Array(array=w390, index=2) -> (element=w391:cluster{string[]})
                n205 = call <vilib>:"NT Read String.vi"("Name"=w393) -> ("String"=w392:string)  [unwired: 9 in, 1 out]
                n206 = Unbundle(w391) -> (w387:string[])
                n207 = Match First String(2:w387, 3:w392) -> (0:w388:i32)  [unwired: 1 out]
                n208 = property on="Test Ring" class="Ring (strict)"("Value"=w388, "Strings []"=w387) -> ()  [unwired: 2 in, 2 out]
                n209 = property on="Test Ring" class="Ring (strict)"("Visible"=TRUE) -> ()  [unwired: 2 in, 2 out]
                n210 = property on="Test Slider" class="Slide (strict)"("Visible"=FALSE) -> ()  [unwired: 2 in, 2 out]
              }
              frame "Exposure Priority  **" {
                n211 = Index Array(array=w399, index=3) -> (element=w400:cluster{string[]})
                n212 = call <vilib>:"NT Read String.vi"("Name"=w402) -> ("String"=w401:string)  [unwired: 9 in, 1 out]
                n213 = Unbundle(w400) -> (w396:string[])
                n214 = Match First String(2:w396, 3:w401) -> (0:w397:i32)  [unwired: 1 out]
                n215 = property on="Test Ring" class="Ring (strict)"("Value"=w397, "Strings []"=w396) -> ()  [unwired: 2 in, 2 out]
                n216 = property on="Test Ring" class="Ring (strict)"("Visible"=TRUE) -> ()  [unwired: 2 in, 2 out]
                n217 = property on="Test Slider" class="Slide (strict)"("Visible"=FALSE) -> ()  [unwired: 2 in, 2 out]
              }
              frame "Color Enable  **" {
                n218 = Index Array(array=w408, index=4) -> (element=w409:cluster{string[]})
                n219 = call <vilib>:"NT Read String.vi"("Name"=w411) -> ("String"=w410:string)  [unwired: 9 in, 1 out]
                n220 = Unbundle(w409) -> (w405:string[])
                n221 = Match First String(2:w405, 3:w410) -> (0:w406:i32)  [unwired: 1 out]
                n222 = property on="Test Ring" class="Ring (strict)"("Value"=w406, "Strings []"=w405) -> ()  [unwired: 2 in, 2 out]
                n223 = property on="Test Ring" class="Ring (strict)"("Visible"=TRUE) -> ()  [unwired: 2 in, 2 out]
                n224 = property on="Test Slider" class="Slide (strict)"("Visible"=FALSE) -> ()  [unwired: 2 in, 2 out]
              }
              frame Default {
                n225 = property on="Test Ring" class="Ring (strict)"("Visible"=FALSE) -> ()  [unwired: 2 in, 2 out]
                n226 = property on="Test Slider" class="Slide (strict)"("Visible"=FALSE) -> ()  [unwired: 2 in, 2 out]
              }
              frame "Brightness  **", "Color Level  **", "Compression  **", "FPS  **", "Sharpness  **" {
                n227 = call <vilib>:"NT Read Number.vi"("Name"=w417) -> ("Numeric"=w416:dbl)  [unwired: 9 in, 1 out]
                n228 = local write "Test Slider"(w416) -> ()
                n229 = property on="Test Slider" class="Slide (strict)"("Visible"=TRUE, "Scale.Maximum"=100.0 ("Scale.Range:Maximum")) -> ()  [unwired: 2 in, 2 out]
                n230 = property on="Test Ring" class="Ring (strict)"("Visible"=FALSE) -> ()  [unwired: 2 in, 2 out]
              }
            }
          }
        }
        n231 = property on="Progress" class="Clust (strict)"("Visible"=FALSE) -> ()  [unwired: 2 in, 2 out]
      }
      event "Test Name": Mouse Enter {
        # "Populate the ring with the list of tests"
        n232 = event-data() -> ()  [unwired: 1 in, 1 out]
        n233 = call <vilib>:"NT Read String Array.vi"("Name"="TestMode/TestList") -> ("String Array"=w425:string[])  [unwired: 9 in, 1 out]
        n234 = Build Array (concatenate)("Select the test to run...", w425) -> (w424:string[])
        n235 = property on="Test Name" class="Ring (strict)"("Strings []"=w424) -> ()  [unwired: 2 in, 2 out]
      }
      event "Test Name": Value Change {
        w427 = FALSE ("Visible")
        # "Tell the robot the test name to run"
        n236 = event-data() -> ("NewVal"=w431:u16)  [unwired: 1 in]
        n237 = property on="Test Name" class="Ring (strict)"() -> ("Strings []"=w432:string[])  [unwired: 2 in, 2 out]
        n238 = local write "Progress"(T9 {"Test Progress"=0, "Test Progress Text"=""} ("Progress")) -> ()
        n239 = Index Array(array=w432, index=w431) -> (element=w430:string)
        n240 = call <vilib>:"NT Write String.vi"("String"=w430, "Name"="TestMode/TestName") -> ()  [unwired: 9 in, 1 out]
        n241 = property on="Progress" class="Clust (strict)"("Visible"=TRUE) -> ()  [unwired: 2 in, 2 out]
        n242 = property on="Motor" class="Clust (strict)"("Visible"=w427) -> ()  [unwired: 2 in, 2 out]
        n243 = property on="Test Slider" class="Slide (strict)"("Visible"=w427) -> ()  [unwired: 2 in, 2 out]
        n244 = property on="On/Off" class="Bool (strict)"("Visible"=w427) -> ()  [unwired: 2 in, 2 out]
        n245 = property on="Rev/Fwd" class="Clust (strict)"("Visible"=w427) -> ()  [unwired: 2 in, 2 out]
        n246 = property on="Test Ring" class="Ring (strict)"("Visible"=w427) -> ()  [unwired: 2 in, 2 out]
      }
      event "DB Camera Config": Value Change {
        n247 = event-data() -> ("NewVal"=w437:bool)  [unwired: 1 in]
        n248 = case shown="False" w437 {
          tunnel: w436 -> [w446 _]
          tunnel: [w439 w457] -> w435
          tunnel: w434 -> [w438 w457]
          frame False {
            w453 = "Camera"
            w456 = FALSE ("Visible")
            n249 = local read "Camera Settings"() -> (w445:T2)
            n250 = Index Array(array=w446) -> (element=w449:cluster{string[]})  [unwired: 1 in]
            n251 = Unbundle(w445) -> ("Frame Rate"=w444:i32, "Compression"=w443:i32, "Size"=w447:u16)
            n252 = Unbundle(w449) -> (w448:string[])
            n253 = Index Array(array=w448, index=w447) -> (element=w442:string)
            n254 = call-poly <vilib>:"Write Key.vi"("section"=w453, "value"=w442, "key"="Size", "refnum"=w438) -> ("refnum out"=w455:T18)  [unwired: 2 in, 5 out]
            n255 = call-poly <vilib>:"Write Key.vi"("section"=w453, "value"=w444, "key"="FrameRate", "refnum"=w455) -> ("refnum out"=w454:T18)  [unwired: 1 in, 6 out]
            n256 = property on="Camera Settings" class="Clust (strict)"("Visible"=w456) -> ()  [unwired: 2 in, 2 out]
            n257 = local write "DB Camera Config"(w456) -> ()
            n258 = call-poly <vilib>:"Write Key.vi"("section"=w453, "value"=w443, "key"="Compression", "refnum"=w454) -> ("refnum out"=w440:T18)  [unwired: 1 in, 6 out]
            n259 = call <vilib>:"Close Config Data.vi"("refnum"=w440) -> ("file path"=w441:path)  [unwired: 2 in, 8 out]
            n260 = call <vilib>:"Open Config Data.vi"("configuration file path"=w441) -> ("refnum"=w439:T18)  [unwired: 8 in, 2 out]
          }
          frame True {
            n261 = property on="Camera Settings" class="Clust (strict)"("Visible"=TRUE) -> ()  [unwired: 2 in, 2 out]
          }
        }
      }
      event "Camera Settings": Value Change {
        n262 = event-data() -> ("NewVal"=w470:T2)  [unwired: 1 in]
        n263 = Index Array(array=w466) -> (element=w465:cluster{string[]})  [unwired: 1 in]
        n264 = Unbundle(w470) -> ("Frame Rate"=w461:i32, "Compression"=w460:i32, "Size"=w463:u16)
        n265 = Unbundle(w465) -> (w464:string[])
        n266 = Index Array(array=w464, index=w463) -> (element=w462:string)
        n267 = Format Into String(format string="%s   %dfps   %d%%", w462, w461, w460) -> (resulting string=w467:string)  [unwired: 2 in, 1 out]
        n268 = Build Array(w467) -> (w468:string[])
        n269 = property on="DB Camera Config" class="Bool (strict)"("Strings [4]"=w468) -> ()  [unwired: 2 in, 2 out]
      }
      event "Motor.Enable": Value Change {
        n270 = event-data() -> ("NewVal"=w476:bool)  [unwired: 1 in]
        n271 = Unbundle("Motor") -> ("Value"=w475:dbl)  [unwired: 1 out]
        n272 = Select(t=w475, s=w476, f=0.0) -> (s? t:f=w473:dbl)
        n273 = call <vilib>:"NT Write Number.vi"("Numeric"=w473, "Name"=w472) -> ()  [unwired: 9 in, 1 out]
      }
      event "Test Slider": Value Change {
        n274 = event-data() -> ("NewVal"=w479:dbl)  [unwired: 1 in]
        n275 = call <vilib>:"NT Write Number.vi"("Numeric"=w479, "Name"=w480) -> ()  [unwired: 9 in, 1 out]
      }
      event "On/Off": Value Change {
        n276 = event-data() -> ("NewVal"=w484:bool)  [unwired: 1 in]
        n277 = Boolean To (0,1)(Boolean=w484) -> (0, 1=w483:i16)
        n278 = call <vilib>:"NT Write Number.vi"("Numeric"=w483, "Name"=w482) -> ()  [unwired: 9 in, 1 out]
      }
      event "Rev/Fwd": Value Change {
        n279 = event-data() -> ("NewVal.Forward"=w492:bool, "NewVal.Reverse"=w491:bool)  [unwired: 1 in]
        n280 = Boolean To (0,1)(Boolean=w492) -> (0, 1=w488:i16)
        n281 = Boolean To (0,1)(Boolean=w491) -> (0, 1=w490:i16)
        n282 = Negate(x=w490) -> (-x=w489:i16)
        n283 = Add(x=w488, y=w489) -> (x+y=w487:i16)
        n284 = call <vilib>:"NT Write Number.vi"("Numeric"=w487, "Name"=w486) -> ()  [unwired: 9 in, 1 out]
      }
      event "Test Ring": Value Change {
        n285 = event-data() -> ("NewVal"=w496:u16)  [unwired: 1 in]
        n286 = property on="Test Ring" class="Ring (strict)"() -> ("Strings []"=w497:string[])  [unwired: 2 in, 2 out]
        n287 = Index Array(array=w497, index=w496) -> (element=w495:string)
        n288 = call <vilib>:"NT Write String.vi"("String"=w495, "Name"=w494) -> ()  [unwired: 9 in, 1 out]
      }
      event "Rec Mode": Value Change {
        # "Update globals for recording mode and path to read log from.\nClear when logging and let NetworkTables set path for vision to\nuse."
        n289 = event-data() -> ("NewVal"=w507:enum32{"Stop", "Record", "Playback"})  [unwired: 1 in]
        n290 = global write "WPI_DashboardLogging Global.vi" "Logging Filename"(path "") -> ()
        n291 = case shown="\"Stop\", \"Record\"" w507 {
          tunnel: w506 -> [_ w509 w517]
          tunnel: [_ _ w516] -> w503
          tunnel: [_ _ w515] -> _
          tunnel: w501 -> [_ _ w513]
          tunnel: cluster{i32, i32} {-250, 170} -> [_ _ w512]
          tunnel: [_ _ T19 {"Image Size"=TRUE, "Image Type"=TRUE, "Pixel Value"=TRUE, "ROI Information"=TRUE, "Zoom Factor"=FALSE} ("Image Information Shown:All Elements")] -> w499
          tunnel: [_ _ TRUE ("Zoom Factor")] -> w498
          frame Default {
          }
          frame "Stop", "Record" {
            # "Place Window too"
            n292 = invoke class="VI" method="FP.Close"(reference=w509) -> (reference out=w508:refnum<vi>)  [unwired: 2 in, 2 out]
            n293 = invoke class="VI" method="Abort VI"(reference=w508) -> ()  [unwired: 2 in, 3 out]
          }
          frame "Playback" {
            n294 = call "Open Playback Panel.vi"("Offset"=w512, "DB VI Ref"=w513, "Playback in"=w517) -> ("Playback out"=w514:refnum<vi>)  [unwired: 8 in]
            n295 = register-events(w514) -> (reference out=w516:refnum<event-registration>, error out=w515:errorcluster)  [unwired: 2 in]
          }
        }
        n296 = global write "WPI_DashboardLogging Global.vi" "Recording"(w507) -> ()
        n297 = property on="Camera Image" class="ImageControl"("Image Information Shown"=w499, "Image Information Visible"=w498) -> ()  [unwired: 2 in, 2 out]
        n298 = call <vilib>:"WPI_DashboardNT Log FieldName Cache.vi"("Operation"=enum16{"Lookup/Add", "Index", "Clear"}."Clear") -> ()  [unwired: 8 in, 3 out]
      }
      event Panel Close {
        w518 = enum32{"Stop", "Record", "Playback"}."Stop" ("Rec Mode")
        n299 = event-data() -> ()  [unwired: 1 in, 4 out]
        n300 = local write "Rec Mode"(w518) -> ()
        n301 = global write "WPI_DashboardLogging Global.vi" "Recording"(w518) -> ()
      }
      event Panel Close {
        # "Abort playback window and ourself"
        n302 = event-data() -> ()  [unwired: 1 in, 4 out]
        n303 = invoke class="VI" method="FP.Close"(reference=w523) -> (reference out=w522:refnum<vi>)  [unwired: 2 in, 2 out]
        n304 = invoke class="VI" method="Abort VI"(reference=w522) -> (error out=w521:errorcluster)  [unwired: 2 in, 2 out]
        n305 = invoke class="VI" method="Abort VI"(error in=w521) -> ()  [unwired: 2 in, 3 out]
      }
    }
  }
  n306 = property on="On/Off" class="Bool (strict)"("Visible"=w27) -> ()  [unwired: 2 in, 2 out]
  n307 = property on="Motor" class="Clust (strict)"("Visible"=w27) -> ()  [unwired: 2 in, 2 out]
  n308 = property on="Progress" class="Clust (strict)"("Visible"=w27) -> ()  [unwired: 2 in, 2 out]
  n309 = property on="Test Ring" class="Ring (strict)"("Visible"=w27) -> ()  [unwired: 2 in, 2 out]
  n310 = property on="Rev/Fwd" class="Clust (strict)"("Visible"=w27) -> ()  [unwired: 2 in, 2 out]
  n311 = property on="Camera Settings" class="Clust (strict)"("Visible"=w27) -> ()  [unwired: 2 in, 2 out]
  n312 = local write "DB Camera Config"(w27) -> ()
  n313 = global write "WPI_DashboardLogging Global.vi" "Recording"(w11) -> ()
  n314 = local write "Rec Mode"(w11) -> ()
